vi "callThread.vi"(0 "HGF_ThreadWorker":refnum<class "HGF_ThreadWorker.lvclass">, 1 "HGF_ThreadPool_Reference":refnum<class "HGF_Reference.lvclass">, 5 "error in (no error)":errorcluster) -> (19 "error out":errorcluster)   [LabVIEW 2014, in "HGF_BaseClasses.lvlib" / "HGF_ThreadWorker.lvclass"]
doc: "call reentrant thread.vi"
uses:
  HGF_ThreadWorker.lvclass
  HGF_Reference/HGF_Reference.lvclass
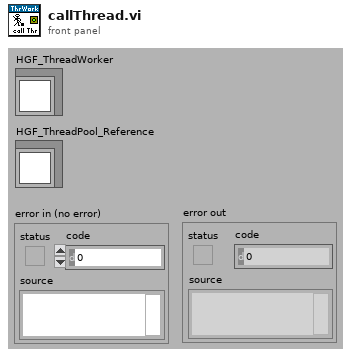
[diagram p1: front panel]
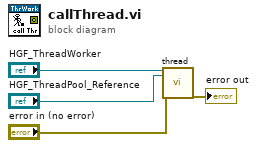
[diagram p0: block diagram]
diagram:
  n1 = call-dynamic "thread.vi"("HGF_ThreadWorker"="HGF_ThreadWorker", "HGF_ThreadPool_Reference"="HGF_ThreadPool_Reference", "error in (no error)"="error in (no error)") -> ("error out"=→"error out":errorcluster)  [unwired: 16 in]
